vi "close_labview.vi"(0 "输入簇":cluster{"载具码":string, "产品码":string, "线号显示":i32}) -> (1 "退出while":bool, 2 "退出Labview":bool)   [LabVIEW 2014]
panel:
  # "外面加延时20ms以及可把时间字符一起"
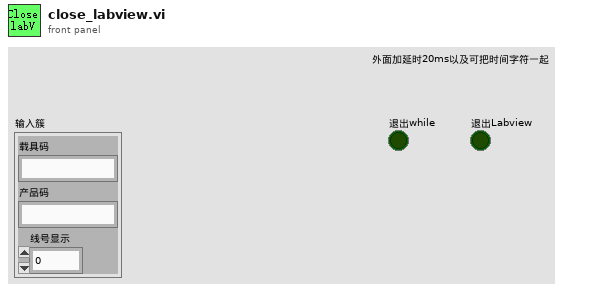
[diagram p1: front panel]
types:
  T1 = enum16{"Left Button", "Center Button", "Right Button", "Window Close"}
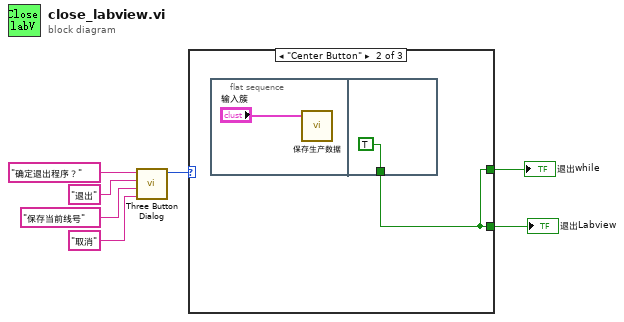
[diagram p0: block diagram]
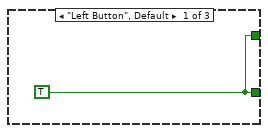
[diagram p2: hidden frame]
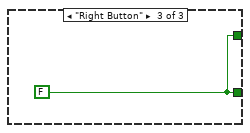
[diagram p3: hidden frame]
diagram:
  n1 = call <vilib>:"Three Button Dialog.vi"("Right Button Text (\"Cancel\")"="取消" ("Right Button Text (\"Cancel\")"), "Center Button Text (\"No\")"="保存当前线号" ("Center Button Text (\"No\")"), "Left Button Text (\"Yes\")"="退出" ("Left Button Text (\"Yes\")"), "message"="确定退出程序？" ("消息")) -> ("Which Button?"=w6:T1)  [unwired: 7 in]
  n2 = case shown="\"Center Button\"" w6 {
    tunnel: [w8 w9 w12] -> w3
    tunnel: [w8 w9 w12] -> w1
    frame "Left Button", Default {
      w8 = TRUE
    }
    frame "Center Button" {
      n3 = flat-sequence {
        tunnel: [TRUE] -> w9
        frame #0 {
          n4 = call "保存生产数据.vi"("输入簇"="输入簇") -> ()  [unwired: 1 in, 1 out]
        }
        frame #1 {
        }
      }
    }
    frame "Right Button" {
      w12 = FALSE
    }
  }
  "退出Labview" <- w3
  "退出while" <- w1
